vi "GetFPS.vi"() -> (0 "FPS":u16)   [LabVIEW 2019]
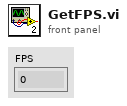
[diagram p1: front panel]
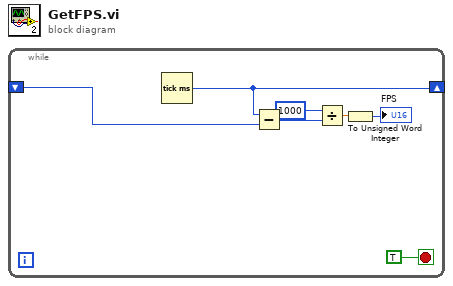
[diagram p0: block diagram]
diagram:
  n1 = while {
    shift-right: [w6] -> _
    shift-left: _ -> [w5]
    stop <- TRUE stop-if-true
    n2 = Tick Count (ms)() -> (millisecond timer value=w6:u32)
    n3 = Subtract(x=w6, y=w5) -> (x-y=w4:u32)
    n4 = Divide(x=u32 1000, y=w4) -> (x/y=w2:dbl)
    n5 = To Unsigned Word Integer(number=w2) -> (unsigned 16bit integer=→"FPS":u16)
  }
